vi "Update Example Control Descriptions.vi"() -> ()   [LabVIEW 2016]
uses:
  <vilib>/Utility/traverseref.llb/TRef TravTarget.ctl
  <vilib>/Utility/traverseref.llb/VI Scripting - Traverse.lvlib
panel:
  in  "Example Directory Path":path=path "../Examples"
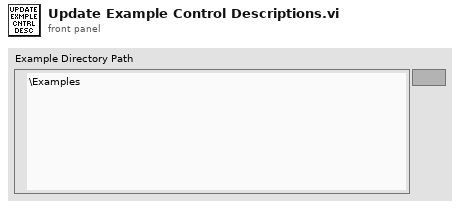
[diagram p1: front panel]
types:
  T1 = typedef "TRef TravTarget.ctl" = enum16{"FP", "BD", "Other"}
  T2 = enum32{"not a typedef", "typedef", "strict typedef", "class private data"}
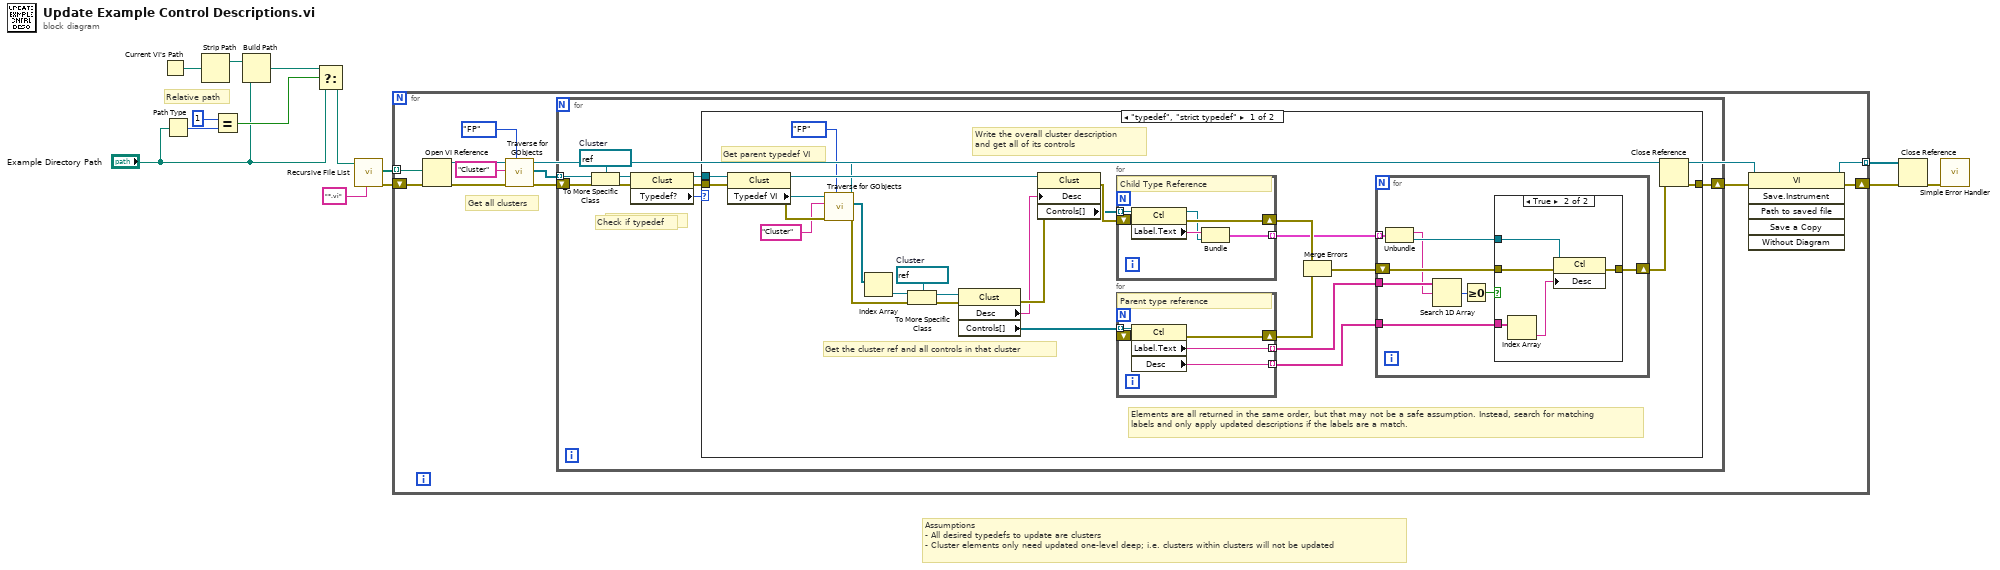
[diagram p0: block diagram]
diagram:
  # "Assumptions\n- All desired typedefs to update are clusters\n- Cluster elements only need updated one-level deep; i.e. clusters within clusters will not be updated"
  # "Relative path"
  n1 = Current VI's Path() -> (path=w9:path)
  n2 = Path Type(1:"Example Directory Path") -> (0:w8:i16)
  n3 = Strip Path(path=w9) -> (stripped path=w6:path)  [unwired: 1 out]
  n4 = Equal?(x=i16 1 ("y"), y=w8) -> (x = y?=w4:bool)
  n5 = Build Path(base path=w6, name or relative path="Example Directory Path") -> (appended path=w5:path)
  n6 = Select(t=w5, s=w4, f="Example Directory Path") -> (s? t:f=w2:path)
  n7 = call <vilib>:"Recursive File List.vi"("pattern"="*.vi", "Folder Path"=w2) -> ("error out"=w13:errorcluster, "All Files in Dir"=w11:path[])  [unwired: 5 in, 3 out]
  n8 = for {
    tunnel: w11 -> [w20] mode=indexing
    shift-right: [w14] -> w10
    shift-left: w13 -> [w24]
    tunnel: [w15] -> w1 mode=indexing
    # "Get all clusters"
    n9 = Open VI Reference(vi path=w20, error in (no error)=w24) -> (vi reference=w18:refnum<vi>, error out=w22:errorcluster)  [unwired: 4 in]
    n10 = call <vilib>:"Traverse for GObjects.vi"("Traverse Target"=TRef_TravTarget."FP", "error in (no error)"=w22, "Class Name"="Cluster", "VI Refnum"=w18) -> ("error out"=w23:errorcluster, "References"=w19:refnum<vi>[])  [unwired: 4 in, 2 out]
    n11 = for {
      tunnel: w19 -> [w27] mode=indexing
      shift-right: [w30] -> w21
      shift-left: w23 -> [w32]
      w25 = refnum<vi> refnum  # Cluster
      # "Check if typedef"
      # "Check if typedef"
      n12 = To More Specific Class(target class=w25, reference=w27, error in=w32) -> (specific class reference=w26:refnum<vi>, error out=w31:errorcluster)
      n13 = property class="Clust"(reference=w26, error in=w31) -> (reference out=w28:refnum<vi>, error out=w33:errorcluster, "Typedef?"=w29:T2)
      n14 = case shown="\"typedef\", \"strict typedef\"" w29 {
        tunnel: w28 -> [w48 _]
        tunnel: w33 -> [w60 w87]
        tunnel: [w59 w87] -> w30
        frame "typedef", "strict typedef" {
          w41 = refnum<vi> refnum  # Cluster
          # "Elements are all returned in the same order, but that may not be a safe assumption. Instead, search for matching labels and only apply updated descriptions if the labels are a match."
          # "Write the overall cluster description and get all of its controls"
          # "Get the cluster ref and all controls in that cluster"
          # "Get parent typedef VI"
          n15 = property class="Clust"(reference=w48, error in=w60) -> (reference out=w46:refnum<vi>, error out=w58:errorcluster, "Typedef VI"=w47:refnum<vi>)
          n16 = call <vilib>:"Traverse for GObjects.vi"("Traverse Target"=TRef_TravTarget."FP", "error in (no error)"=w58, "Class Name"="Cluster", "VI Refnum"=w47) -> ("error out"=w57:errorcluster, "References"=w49:refnum<vi>[], "dup VI Refnum"=w45:refnum<vi>)  [unwired: 4 in, 1 out]
          n17 = Index Array(array=w49) -> (element=w43:refnum<vi>)  [unwired: 1 in]
          n18 = To More Specific Class(target class=w41, reference=w43, error in=w57) -> (specific class reference=w42:refnum<vi>, error out=w56:errorcluster)
          n19 = property class="Clust"(reference=w42, error in=w56) -> (error out=w50:errorcluster, "Desc"=w40:string, "Controls[]"=w38:refnum<vi>[])  [unwired: 1 out]
          n20 = property class="Clust"(reference=w46, error in=w50, "Desc"=w40) -> (error out=w55:errorcluster, "Controls[]"=w39:refnum<vi>[])  [unwired: 1 out]
          n21 = for {
            tunnel: w39 -> [w84] mode=indexing
            shift-right: [w85] -> w54
            shift-left: w55 -> [w86]
            tunnel: [w82] -> w36 mode=indexing
            # "Child Type Reference"
            n22 = property class="Ctl"(reference=w84, error in=w86) -> (reference out=w81:refnum<vi>, error out=w85:errorcluster, "Label.Text"=w83:string)
            n23 = Bundle("Label.Text"=w83, w81) -> (w82:cluster{"Label.Text":string, refnum<vi>})  [unwired: 1 in]
          }
          n24 = for {
            tunnel: w38 -> [w78] mode=indexing
            shift-right: [w79] -> w53
            shift-left: _ -> [w80]
            tunnel: [w77] -> w35 mode=indexing
            tunnel: [w76] -> w34 mode=indexing
            # "Parent type reference"
            n25 = property class="Ctl"(reference=w78, error in=w80) -> (error out=w79:errorcluster, "Label.Text"=w77:string, "Desc"=w76:string)  [unwired: 1 out]
          }
          n26 = Merge Errors(w54, w53) -> (w52:errorcluster)
          n27 = for {
            shift-right: [w69] -> w51
            shift-left: w52 -> [w68]
            tunnel: w36 -> [w65] mode=indexing
            tunnel: w35 -> [w63]
            tunnel: w34 -> [w61]
            n28 = Unbundle(w65) -> ("Label.Text"=w62:string, w64:refnum<vi>)
            n29 = Search 1D Array(1D array=w63, element=w62) -> (index of element=w66:i32)  [unwired: 1 in]
            n30 = Greater Or Equal To 0?(x=w66) -> (x >= 0?=w67:bool)
            n31 = case shown="True" w67 {
              tunnel: [w70 w75] -> w69
              tunnel: w68 -> [w70 w74]
              tunnel: w64 -> [_ w73]
              tunnel: w61 -> [_ w72]
              frame False {
              }
              frame True {
                n32 = Index Array(array=w72) -> (element=w71:string)  [unwired: 1 in]
                n33 = property class="Ctl"(reference=w73, error in=w74, "Desc"=w71) -> (error out=w75:errorcluster)  [unwired: 1 out]
              }
            }
          }
          n34 = Close Reference(reference=w45, error in (no error)=w51) -> (error out=w59:errorcluster)
        }
        frame Default {
        }
      }
    }
    n35 = invoke class="VI" method="Save.Instrument"(reference=w18, error in=w21) -> (reference out=w15:refnum<vi>, error out=w14:errorcluster)  [unwired: 4 in, 4 out]
  }
  n36 = Close Reference(reference=w1) -> ()  [unwired: 1 in, 1 out]
  n37 = call <vilib>:"Simple Error Handler.vi"("error in (no error)"=w10) -> ()  [unwired: 4 in, 5 out]
